vi "Get Control Panel Data.vi"(8 "error in (no error)":errorcluster, 11 "Device in":refnum<class "Device.lvclass">) -> (0 "error out":errorcluster, 2 "Data":variant, 3 "Device out":refnum<class "Device.lvclass">)   [LabVIEW 2015, in "Device.lvclass"]
uses:
  Device.lvclass
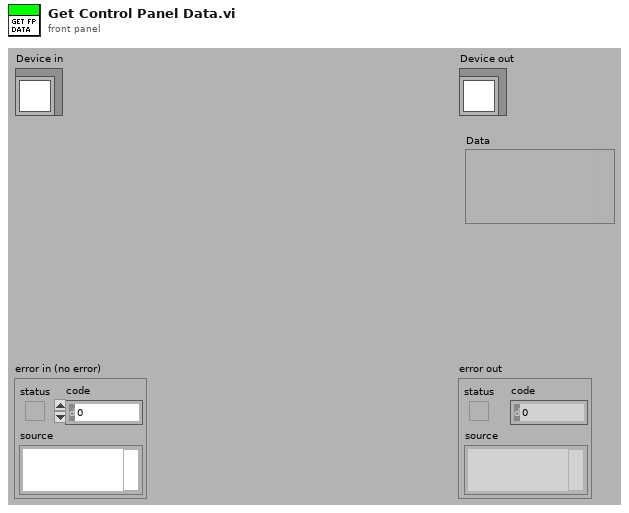
[diagram p1: front panel]
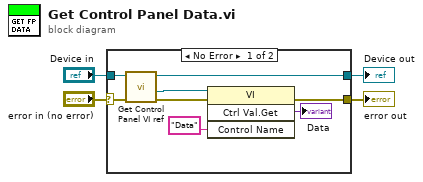
[diagram p0: block diagram]
diagram:
  n1 = case shown="No Error" "error in (no error)" {
    selector: "error in (no error)" -> [w8 w14]
    tunnel: [w5 w14] -> w3
    tunnel: [w11 w13] -> w1
    tunnel: "Device in" -> [w12 w13]
    frame No Error {
      n2 = call "Get Control Panel VI ref.vi"("error in (no error)"=w8, "Device in"=w12) -> ("error out"=w9:errorcluster, "vi ref out"=w10:refnum<vi>, "Device out"=w11:refnum<class "Device.lvclass">)  [unwired: 7 in]
      n3 = invoke class="VI" method="Ctrl Val.Get"(reference=w10, error in=w9, "Control Name"="Data") -> (error out=w5:errorcluster, "Get Control Value Variant"=→"Data":variant)  [unwired: 1 in, 2 out]
    }
    frame Error {
    }
  }
  "error out" <- w3
  "Device out" <- w1
